vi "Loop Get FeedbackNode Init Terminals.vi"(11 "GObject in":refnum<vi>) -> (3 "feedback nodes init terms[]":refnum<vi>[](array[refnum]))   [LabVIEW 2018]
doc: "Returns referencies to initialize terminals of feedback inside loop which have set initialize terminal outside loop."
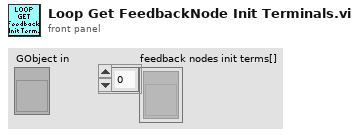
[diagram p1: front panel]
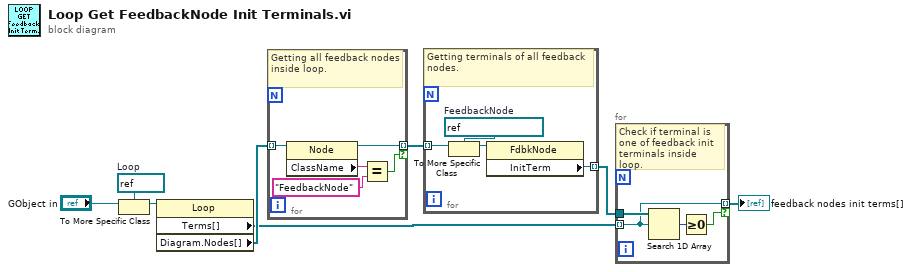
[diagram p0: block diagram]
diagram:
  w2 = refnum<vi> refnum  # Loop
  n1 = To More Specific Class(target class=w2, reference="GObject in") -> (specific class reference=w3:refnum<vi>)  [unwired: 1 in, 1 out]
  n2 = property class="Loop"(reference=w3) -> ("Terms[]"=w4:refnum<vi>[], "Diagram.Nodes[]"=w5:refnum<vi>[])  [unwired: 1 in, 2 out]
  n3 = for {
    tunnel: w5 -> [w13] mode=indexing
    tunnel: [w10] -> w6 mode=indexing if=w9
    # "Getting all feedback nodes inside loop."
    n4 = property class="Node"(reference=w13) -> (reference out=w10:refnum<vi>, "ClassName"=w12:string)  [unwired: 1 in, 1 out]
    n5 = Equal?(x=w12, y="FeedbackNode") -> (x = y?=w9:bool)
  }
  n6 = for {
    tunnel: w6 -> [w17] mode=indexing
    tunnel: [w14] -> w7 mode=indexing
    w16 = refnum<vi> refnum  # FeedbackNode
    # "Getting terminals of all feedback nodes."
    n7 = To More Specific Class(target class=w16, reference=w17) -> (specific class reference=w15:refnum<vi>)  [unwired: 1 in, 1 out]
    n8 = property class="FdbkNode"(reference=w15) -> ("InitTerm"=w14:refnum<vi>)  [unwired: 1 in, 2 out]
  }
  n9 = for {
    tunnel: w4 -> [w18] mode=indexing
    tunnel: [w18] -> w8 mode=indexing if=w19
    tunnel: w7 -> [w21]
    # "Check if terminal is one of feedback init terminals inside loop."
    n10 = Search 1D Array(1D array=w21, element=w18) -> (index of element=w20:i32)  [unwired: 1 in]
    n11 = Greater Or Equal To 0?(x=w20) -> (x >= 0?=w19:bool)
  }
  "feedback nodes init terms[]" <- w8
